vi "Record (Save to Log Data File).vi"(0 "Start/Stop Recording In":bool, 1 "Formatted Data String In":string, 2 "Recording State (Previous Loop) In":bool, 3 "Record File Refnum In":refnum<file>, 4 "Last Recording Filename In":string, 5 "Error In":errorcluster) -> (6 "Record File Refnum Out":refnum<file>, 7 "Error Out":errorcluster, 8 "Last Recording Filename Out":string)   [LabVIEW 2020]
doc: "Record (Save to Log Data File).vi prompts the user for a file path, name, and type when recording starts, adds a header to the file, and logs the formatted data string to the file each iteration until Start/Stop Recording is FALSE."
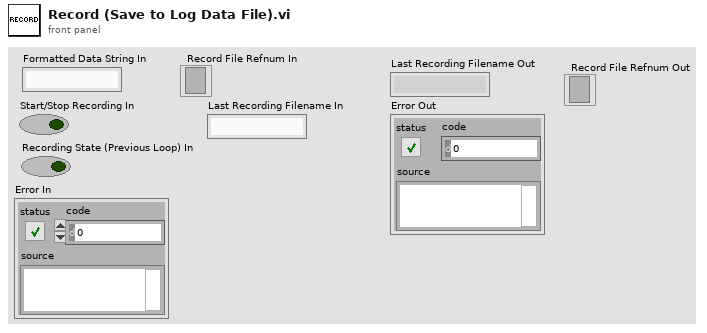
[diagram p1: front panel]
types:
  T1 = enum16{"open", "replace", "create", "open or create", "replace or create", "replace or create with confirmation"}
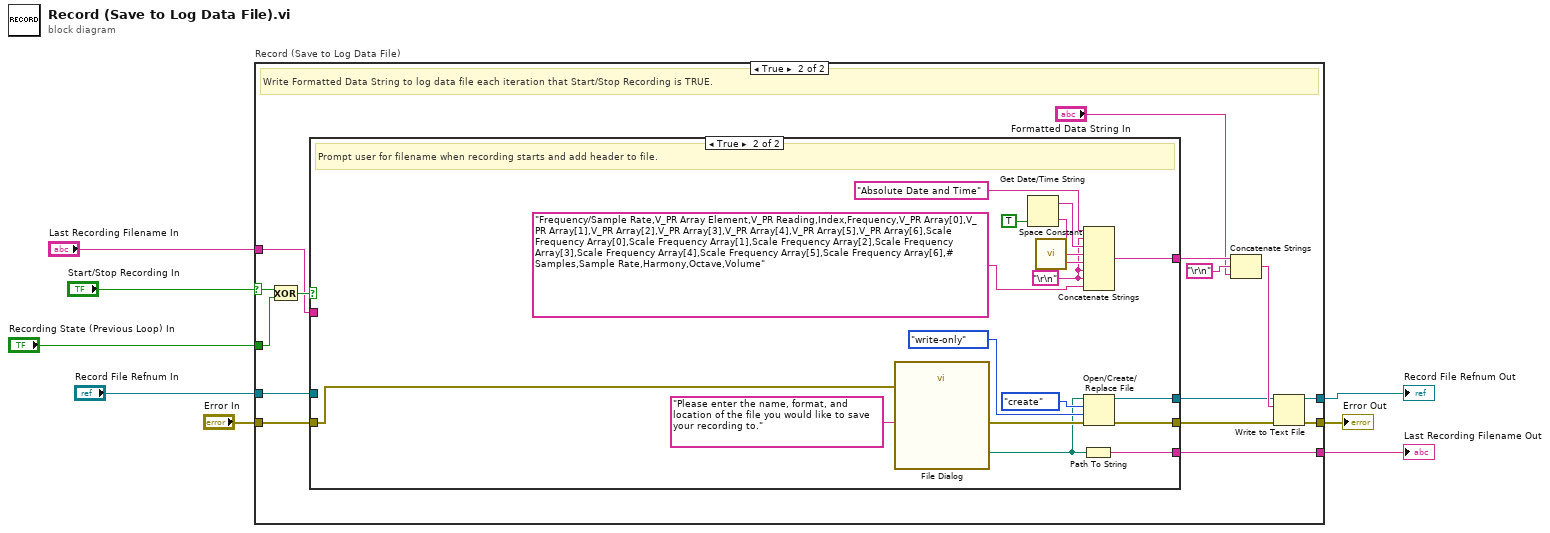
[diagram p0: block diagram]
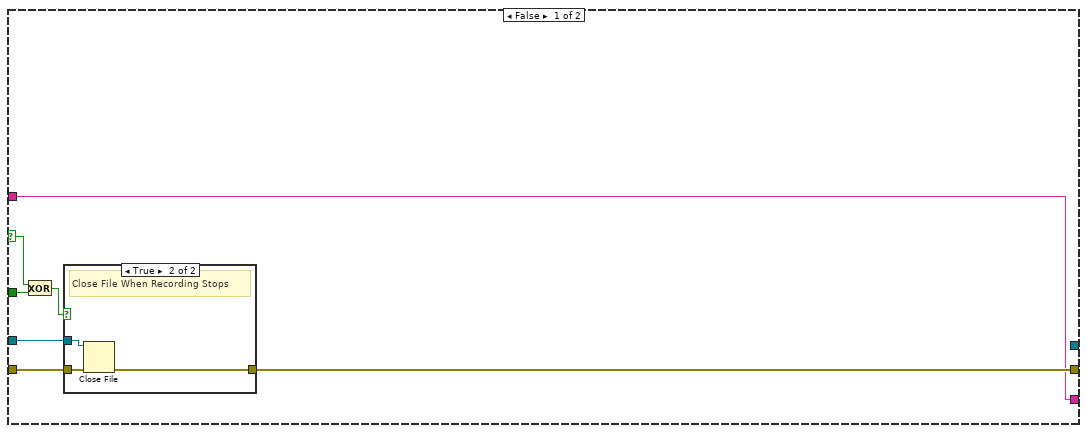
[diagram p2: hidden frame]
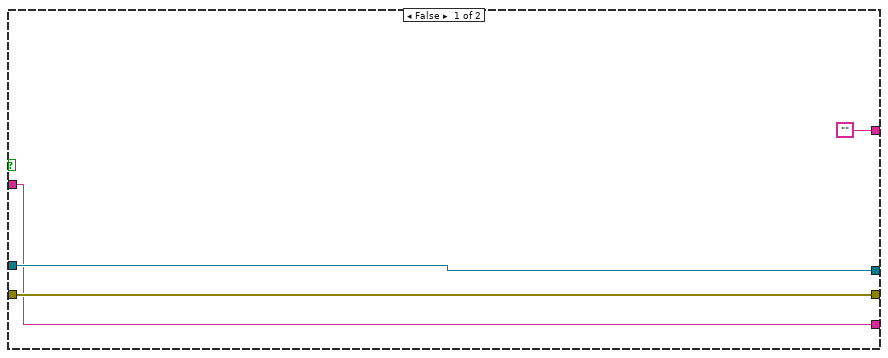
[diagram p4: hidden frame]
diagram:
  n1 = case "Record (Save to Log Data File)" shown="True" "Start/Stop Recording In" {
    selector: "Start/Stop Recording In" -> [w15 w34]
    tunnel: "Recording State (Previous Loop) In" -> [w14 w33]
    tunnel: [_ w29] -> w1
    tunnel: "Record File Refnum In" -> [w12 w28]
    tunnel: [w11 w30] -> w2
    tunnel: "Error In" -> [w10 w26]
    tunnel: [w9 w24] -> w3
    tunnel: "Last Recording Filename In" -> [w9 w23]
    frame False {
      n2 = Exclusive Or(1:w14, 2:w15) -> (0:w13:bool)
      n3 = case shown="True" w13 {
        tunnel: w12 -> [_ w19]
        tunnel: [w16 w18] -> w11
        tunnel: w10 -> [w16 w17]
        frame False {
        }
        frame True {
          # "Close File When Recording Stops"
          n4 = Close File(refnum=w19, error in=w17) -> (error out=w18:errorcluster)  [unwired: 1 out]
        }
      }
    }
    frame True {
      # "Write Formatted Data String to log data file each iteration that Start/Stop Recording is TRUE."
      n5 = Exclusive Or(1:w33, 2:w34) -> (0:w32:bool)
      n6 = case shown="True" w32 {
        tunnel: [w37 w51] -> w31
        tunnel: [w38 w50] -> w25
        tunnel: w28 -> [w38 _]
        tunnel: w26 -> [w37 w49]
        tunnel: [w36 w47] -> w24
        tunnel: w23 -> [w36 _]
        tunnel: ["" w41] -> w22
        frame False {
        }
        frame True {
          w39 = "\r\n"
          # "Prompt user for filename when recording starts and add header to file."
          n7 = call "File Dialog"("prompt"="Please enter the name, format, and location of the file you would like to save your recording to.", "error in"=w49) -> ("selected path"=w48:path, "error out"=w52:errorcluster)  [unwired: 10 in, 2 out]
          n8 = Get Date/Time String(want seconds? (F)=TRUE) -> (date string=w44:string, time string=w42:string)  [unwired: 2 in]
          n9 = call <vilib>:"Space Constant.vi"() -> ("String"=w43:string)
          n10 = Path To String(path=w48) -> (string=w47:string)
          n11 = Concatenate Strings("Absolute Date and Time" ("string"), w39, w44, w43, w42, w39, w39, "Frequency/Sample Rate,V_PR Array Element,V_PR Reading,Index,Frequency,V_PR Array[0],V_PR Array[1],V_PR Array[2],V_PR Array[3],V_PR Array[4],V_PR Array[5],V_PR Array[6],Scale Frequency Array[0],Scale Frequency Array[1],Scale Frequency Array[2],Scale Frequency Array[3],Scale Frequency Array[4],Scale Frequency Array[5],Scale Frequency Array[6],# Samples,Sample Rate,Harmony,Octave,Volume" ("string")) -> (w41:string)
          n12 = Open/Create/Replace File(file path (use dialog)=w48, error in=w52, operation (0:open)=T1."create", access (0:read/write)=enum16{"read/write", "read-only", "write-only"}."write-only") -> (refnum out=w50:refnum<file>, error out=w51:errorcluster)  [unwired: 2 in, 1 out]
        }
      }
      n13 = Concatenate Strings(w22, "\r\n", "Formatted Data String In") -> (w27:string)
      n14 = Write to Text File(file (use dialog)=w25, text=w27, error in=w31) -> (refnum out=w29:refnum<file>, error out=w30:errorcluster)  [unwired: 1 in, 1 out]
    }
  }
  "Last Recording Filename Out" <- w3
  "Error Out" <- w2
  "Record File Refnum Out" <- w1
